vi "6-Lower&UpperCase.vi"() -> ()   [LabVIEW 2020]
panel:
  out "Length of String":i32
  out "Switched String":string
  in  "Input String":string
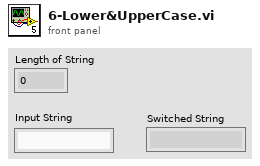
[diagram p1: front panel]
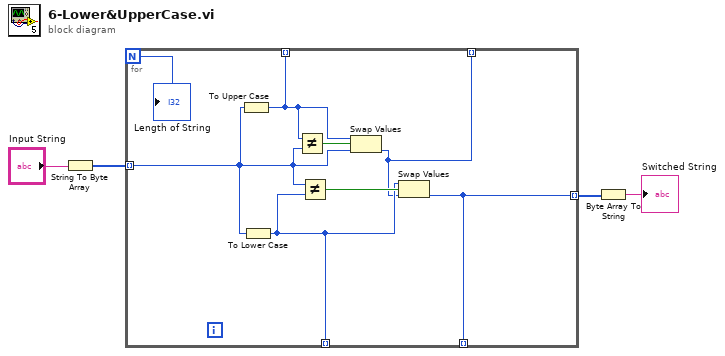
[diagram p0: block diagram]
diagram:
  n1 = String To Byte Array(string="Input String") -> (unsigned byte array=w3:u8[])
  n2 = for {
    N -> [w5]
    tunnel: w3 -> [w10] mode=indexing
    tunnel: [w7] -> w2 mode=indexing
    tunnel: [w9] -> _ mode=indexing
    tunnel: [w8] -> _ mode=indexing
    tunnel: [w7] -> _ mode=indexing
    tunnel: [w6] -> _ mode=indexing
    n3 = To Upper Case(1:w10) -> (0:w9:u8)
    n4 = To Lower Case(string=w10) -> (all lower case string=w8:u8)
    n5 = Not Equal?(x=w9, y=w10) -> (x != y?=w12:bool)
    n6 = Not Equal?(x=w10, y=w8) -> (x != y?=w11:bool)
    n7 = Swap Values(12:w9, 13:w12, 14:w10) -> (3:w6:u8)  [unwired: 1 out]
    n8 = Swap Values(12:w8, 13:w11, 14:w6) -> (3:w7:u8)  [unwired: 1 out]
    "Length of String" <- w5
  }
  n9 = Byte Array To String(unsigned byte array=w2) -> (string=→"Switched String":string)
